vi "Receive I32 Value Msg.vi"(8 "error in (no error)":errorcluster, 10 "I32ValueMsg":refnum<class "I32ValueMsg.lvclass">, 11 "IController In":refnum<class "IController.lvclass">) -> (0 "error out":errorcluster, 3 "IController Out":refnum<class "IController.lvclass">)   [LabVIEW 2015, in "IController.lvlib" / "IController.lvclass"]
uses:
  IController.lvclass
  AutoRegistration/ActorAutoRegistration Messages/I32ValueMsg/I32ValueMsg.lvclass
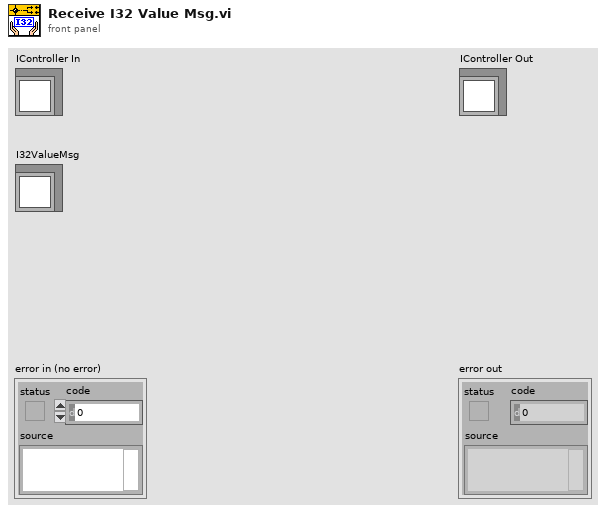
[diagram p1: front panel]
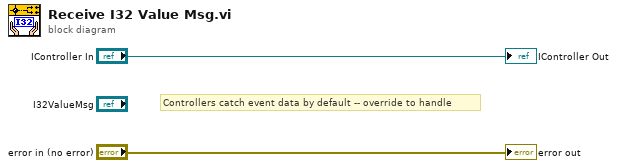
[diagram p0: block diagram]
diagram:
  # "Controllers catch event data by default -- override to handle"
  "error out" <- "error in (no error)"
  "IController Out" <- "IController In"
